vi "Entrenamiento Fuerza 4.vi"(8 "error in (no error)":errorcluster) -> (0 "error out":errorcluster, 3 "Message":string)   [LabVIEW 2014]
panel:
  in  "index":i32
  out "size(s)":i32
  out "Decorations[]":refnum<vi>[](array[refnum])
  out "Boolean":bool
  out "Impulso":string
  out "Tiempo Restante":string
  out "Time Target (s)":dbl=50.0
  out "Tiempo Transcurrido":string
  in  "Start":bool
  in  "Impulso":bool
  in  "Reset":bool
  in  "Back":bool
  in  "Help":bool
  in  "Slider":i32(slide) scale=0.0..100.0
  out "Horizontal Graduated Bar":i16(slide) scale=0.0..100.0
  in  "Remove Button":bool
  in  "Add Button":bool
  out "Opcional %":string="0%"
  in  "Opcional Bool":bool
  out "Biceps %":string="0%"
  in  "Biceps Bool":bool
  out "Pectorales %":string="0%"
  in  "Pectorales Bool":bool
  out "Trapecio %":string="0%"
  in  "Trapecio Bool":bool
  out "Dorsales %":string="0%"
  in  "Dorsales Bool":bool
  out "Lumbares %":string="0%"
  in  "Lumbares Bool":bool
  out "Abdomen %":string="0%"
  in  "Abdomen Bool":bool
  out "Gluteos %":string="0%"
  in  "Gluteos Bool":bool
  out "Isquiotibiales %":string="0%"
  in  "Isquiotibiales Bool":bool
  in  "Stop":bool
  out "Cuadríceps %":string="0%"
  in  "Cuadriceps Bool":bool
  out "date/time string":string="22/08/2015 01:25:29 a. m."
  # "Entrenamiento de Fuerza"
  # "Presentación"
  # "Seg"
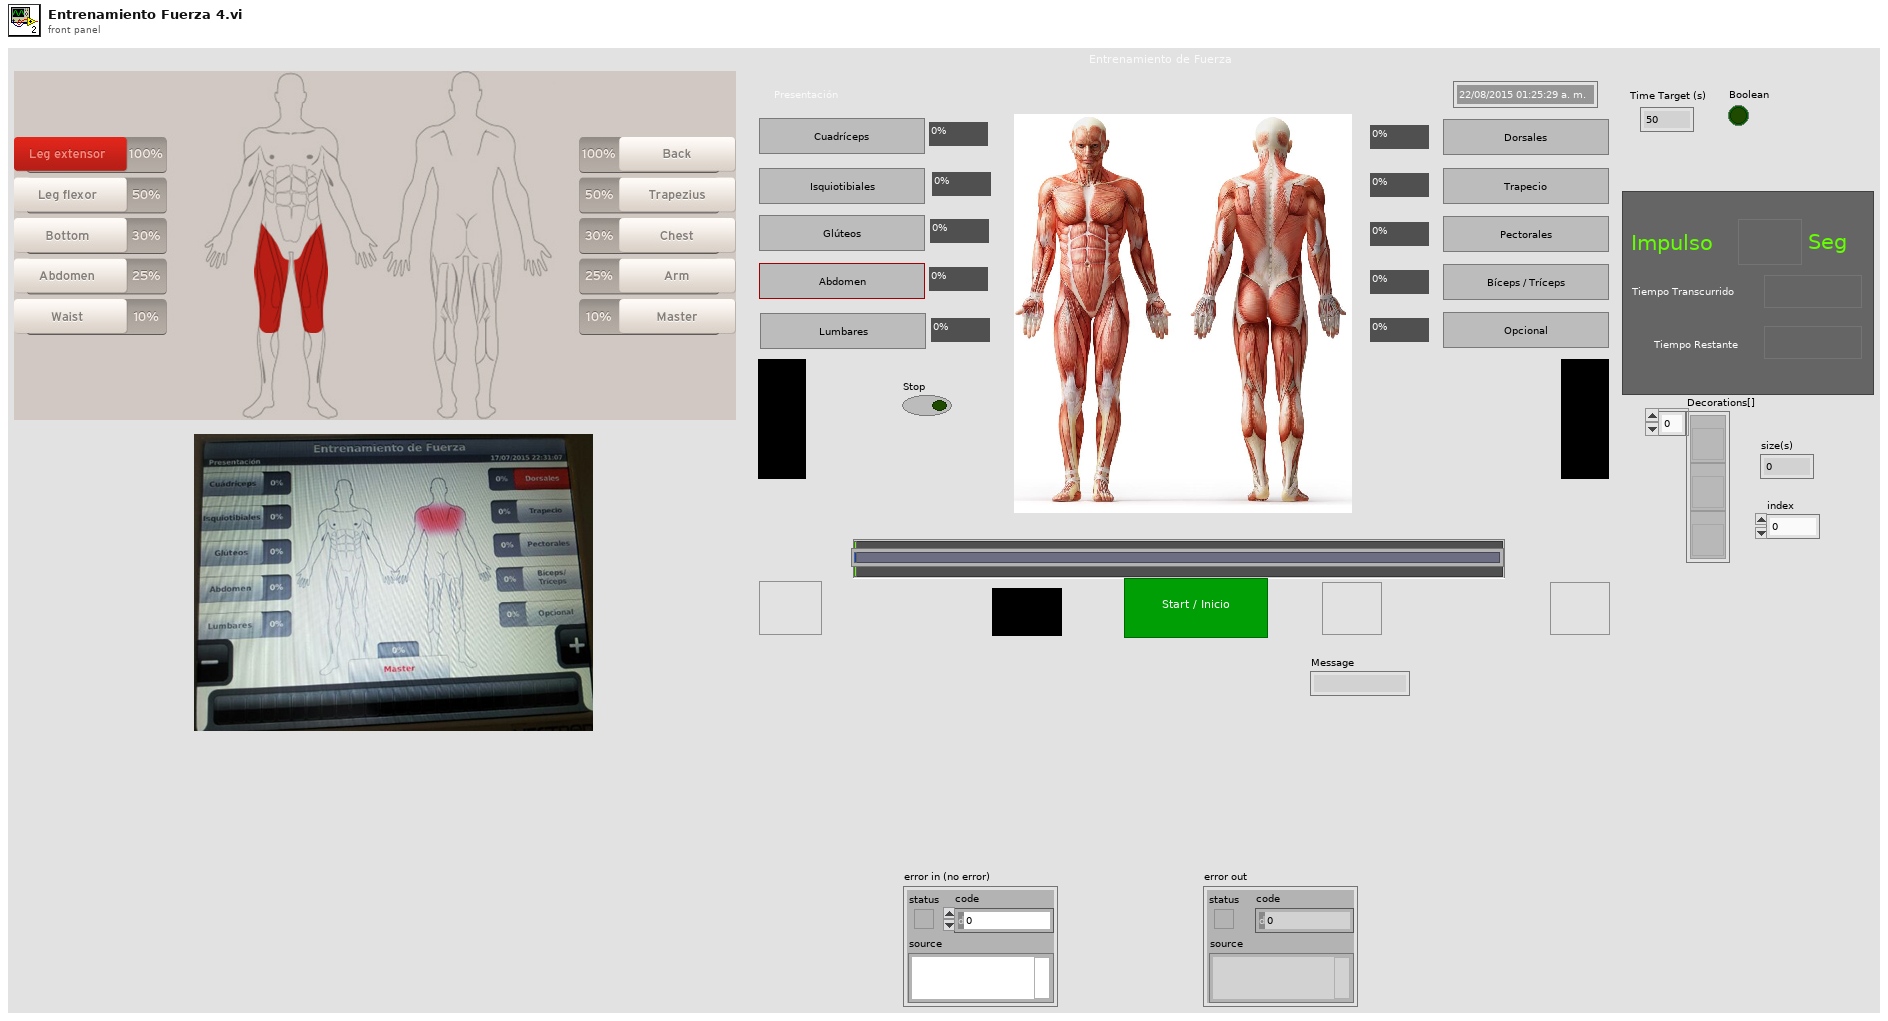
[diagram p1: front panel]
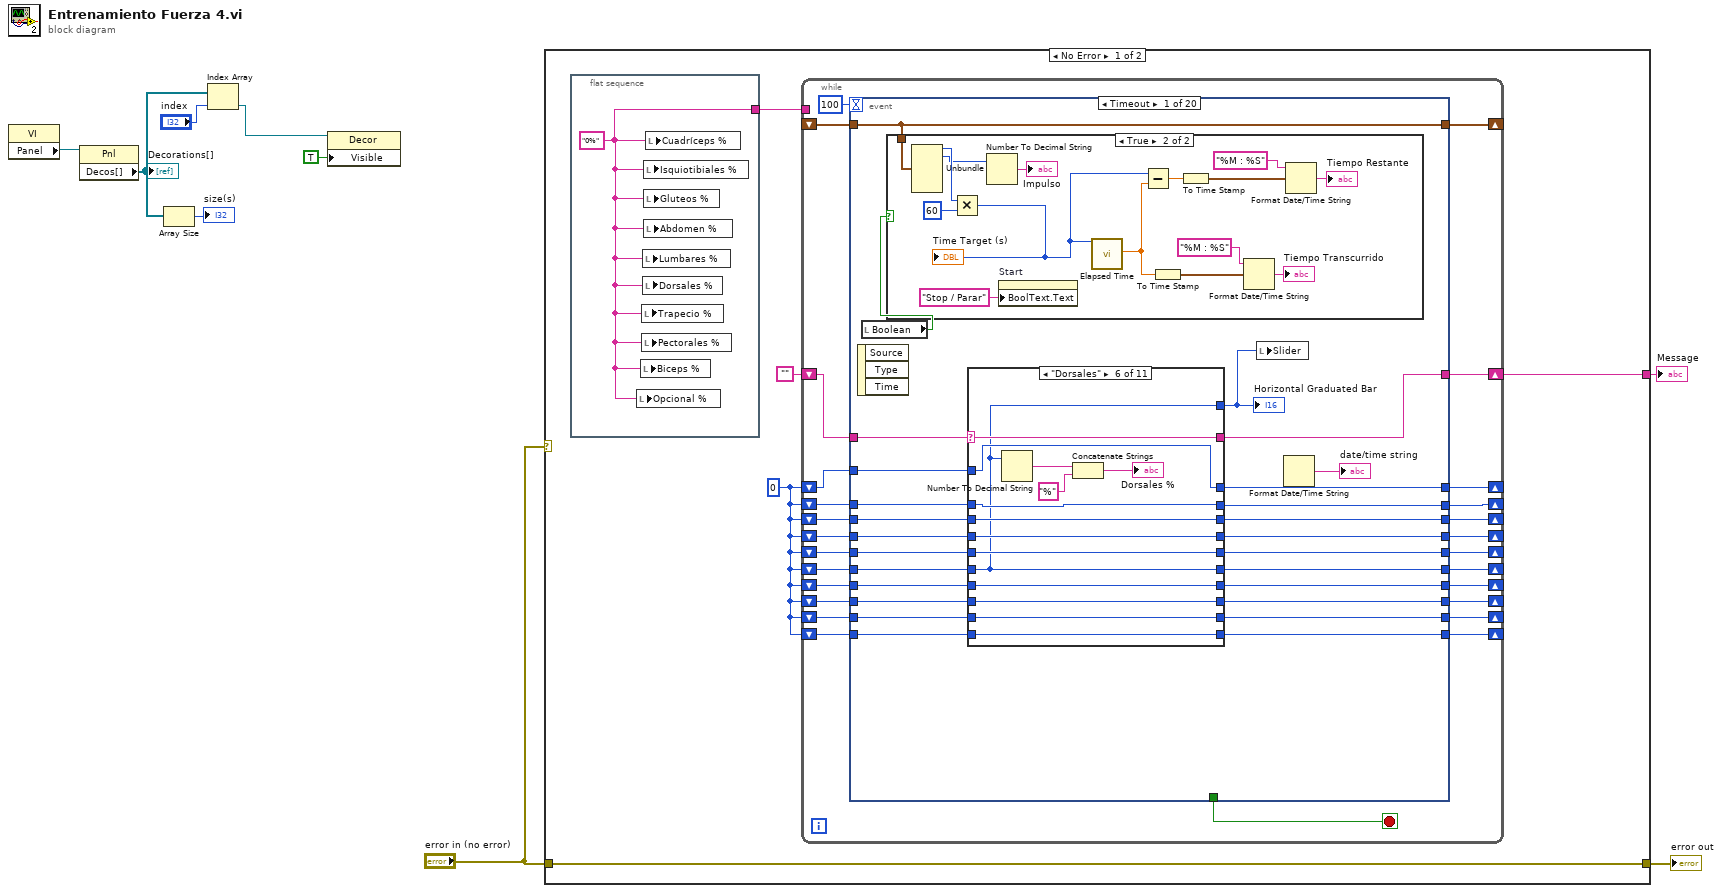
[diagram p0: block diagram]
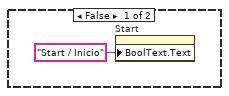
[diagram p2: hidden frame]
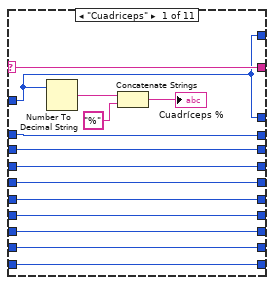
[diagram p3: hidden frame]
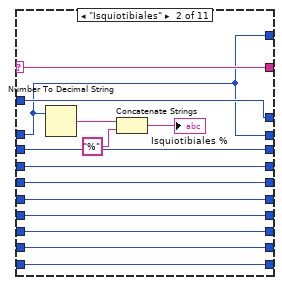
[diagram p4: hidden frame]
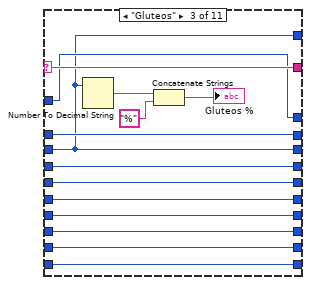
[diagram p5: hidden frame]
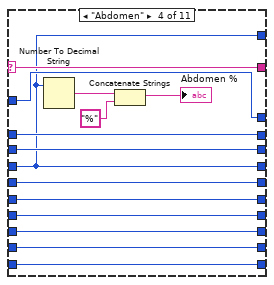
[diagram p6: hidden frame]
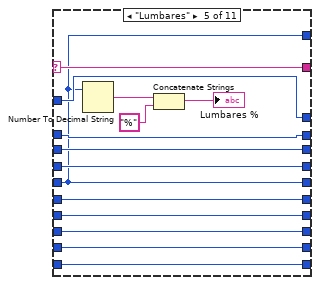
[diagram p7: hidden frame]
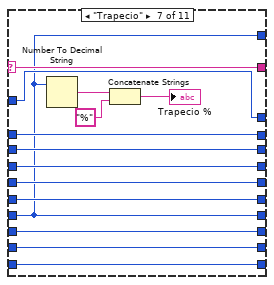
[diagram p8: hidden frame]
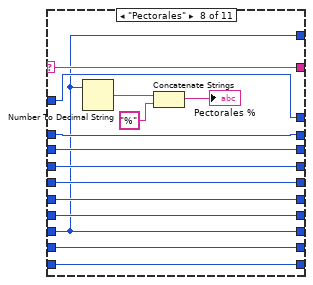
[diagram p9: hidden frame]
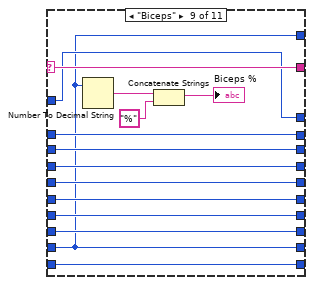
[diagram p10: hidden frame]
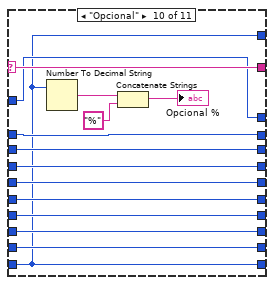
[diagram p11: hidden frame]
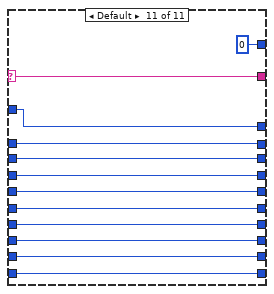
[diagram p12: hidden frame]
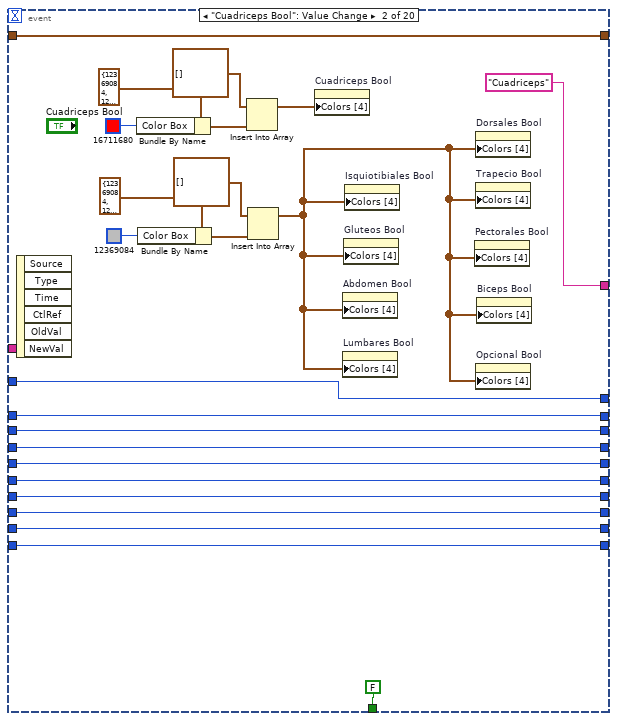
[diagram p13: hidden frame]
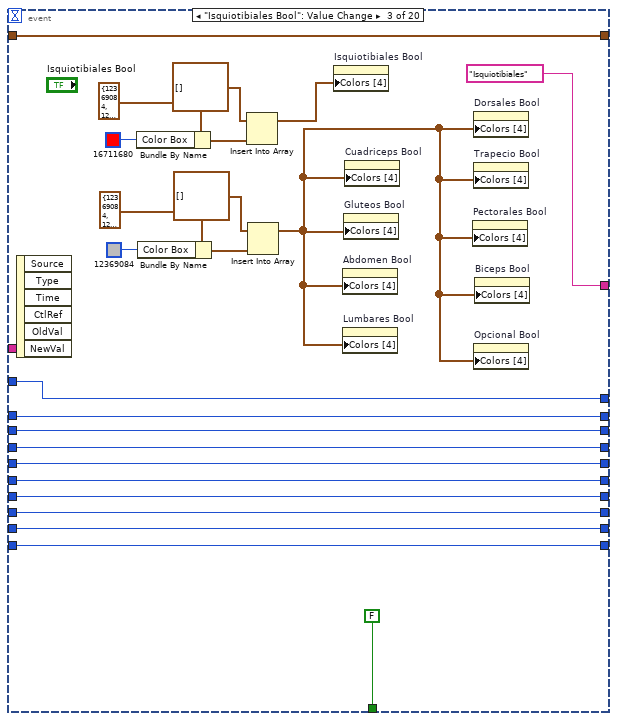
[diagram p14: hidden frame]
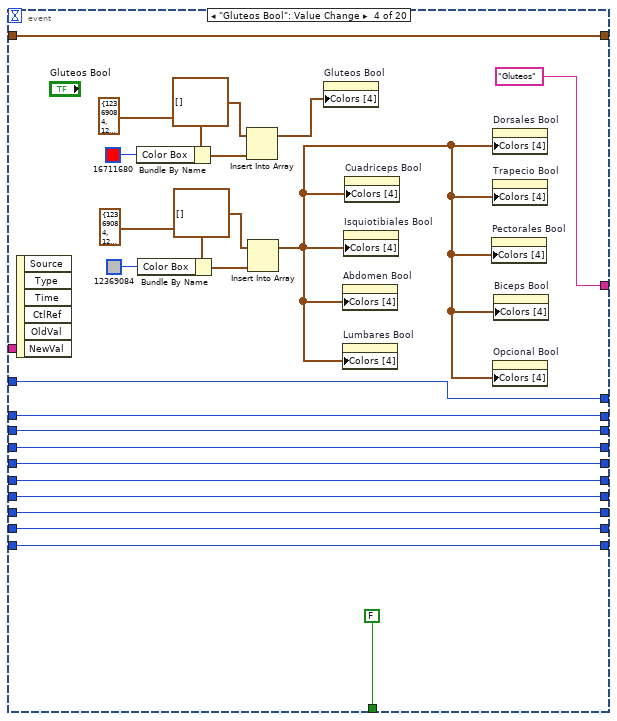
[diagram p15: hidden frame]
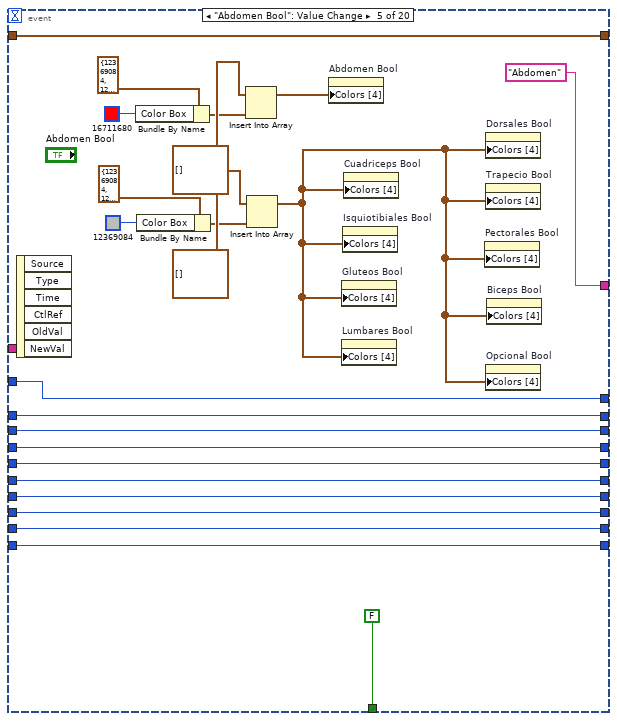
[diagram p16: hidden frame]
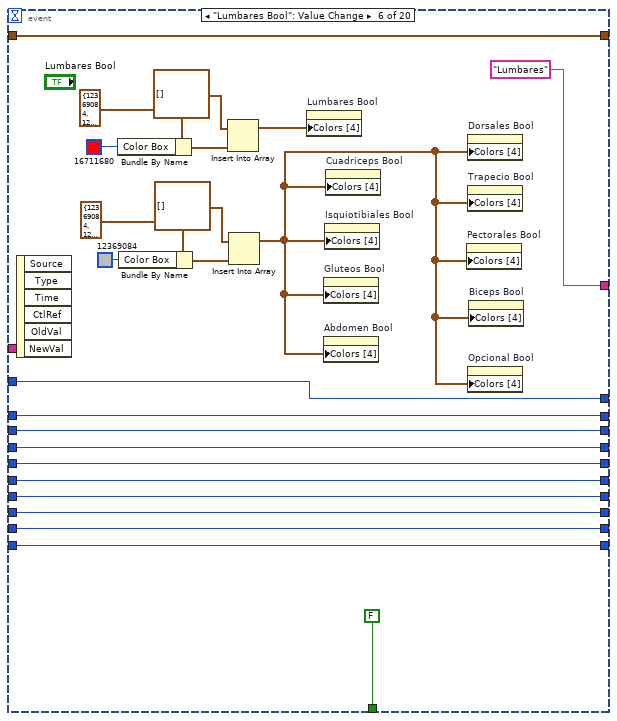
[diagram p17: hidden frame]
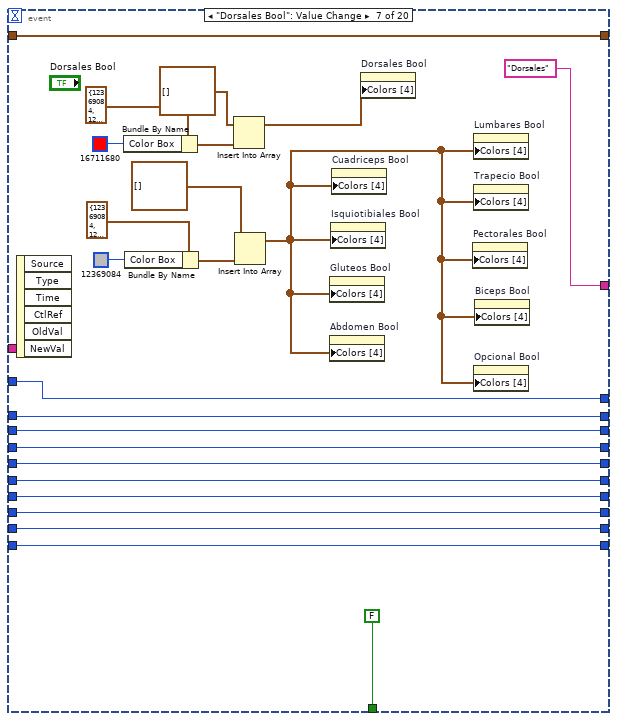
[diagram p18: hidden frame]
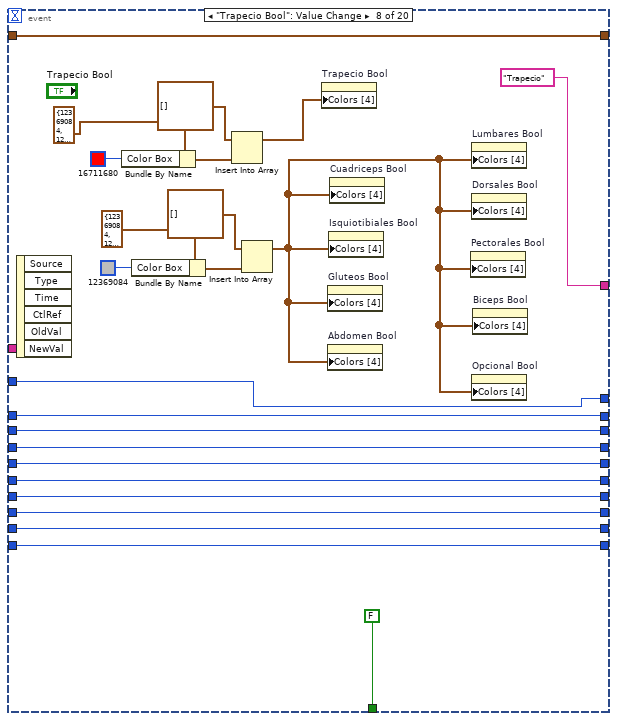
[diagram p19: hidden frame]
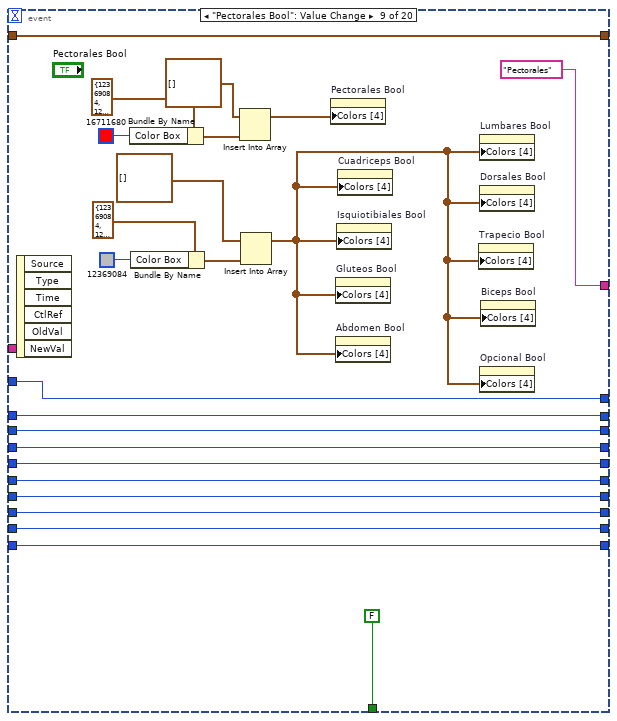
[diagram p20: hidden frame]
diagram:
  n1 = property class="VI"() -> ("Panel"=w6:refnum<vi>)  [unwired: 2 in, 2 out]
  n2 = property class="Pnl"(reference=w6) -> ("Decos[]"=w3:refnum<vi>[])  [unwired: 1 in, 2 out]
  "Decorations[]" <- w3
  n3 = Array Size(array=w3) -> (size(s)=→"size(s)":i32)
  n4 = Index Array(array=w3, index="index") -> (element=w2:refnum<vi>)
  n5 = property class="Decor"(reference=w2, "Visible"=TRUE) -> ()  [unwired: 1 in, 2 out]
  n6 = case shown="No Error" "error in (no error)" {
    tunnel: "error in (no error)" -> [w14 w1043]
    tunnel: [w14 w1043] -> w8
    tunnel: [w13 "Error" ("Message")] -> w7
    frame No Error {
      w11 = 0
      n7 = flat-sequence {
        tunnel: [w15] -> w10
        frame #0 {
          w15 = "0%" ("Cuadríceps %")
          n8 = local write "Opcional %"(w15) -> ()
          n9 = local write "Biceps %"(w15) -> ()
          n10 = local write "Trapecio %"(w15) -> ()
          n11 = local write "Pectorales %"(w15) -> ()
          n12 = local write "Lumbares %"(w15) -> ()
          n13 = local write "Dorsales %"(w15) -> ()
          n14 = local write "Isquiotibiales %"(w15) -> ()
          n15 = local write "Gluteos %"(w15) -> ()
          n16 = local write "Abdomen %"(w15) -> ()
          n17 = local write "Cuadríceps %"(w15) -> ()
        }
      }
      n18 = while {
        shift-right: [w39] -> w13
        shift-left: "" ("Message") -> [w38]
        shift-right: [w18] -> _
        shift-left: w11 -> [w37]
        shift-right: [w19] -> _
        shift-left: w11 -> [w36]
        shift-right: [w20] -> _
        shift-left: w11 -> [w35]
        shift-right: [w21] -> _
        shift-left: w11 -> [w34]
        shift-right: [w22] -> _
        shift-left: w11 -> [w33]
        shift-right: [w23] -> _
        shift-left: w11 -> [w32]
        shift-right: [w24] -> _
        shift-left: w11 -> [w31]
        shift-right: [w25] -> _
        shift-left: w11 -> [w30]
        shift-right: [w26] -> _
        shift-left: w11 -> [w29]
        shift-right: [w27] -> _
        shift-left: w11 -> [w28]
        tunnel: w10 -> [_]
        shift-right: [w16] -> _
        shift-left: _ -> [w17]
        stop <- w41 stop-if-true
        n19 = event shown="[0] Timeout" {
          selector: _ -> [_ _ _ _ _ _ _ _ _ _ _ _ _ _ _ _ _ _ _ _]
          dyn-events: _ -> [_ _ _ _ _ _ _ _ _ _ _ _ _ _ _ _ _ _ _ _]
          timeout: 100 -> [_ _ _ _ _ _ _ _ _ _ _ _ _ _ _ _ _ _ _ _]
          tunnel: [_ FALSE FALSE FALSE FALSE FALSE FALSE FALSE FALSE FALSE FALSE _ _ _ "Stop" TRUE ("Stop") FALSE ("Stop") TRUE ("Stop") FALSE ("Stop") _] -> w41
          tunnel: [w65 "Cuadriceps" ("Message") "Isquiotibiales" ("Message") "Gluteos" ("Message") "Abdomen" ("Message") "Lumbares" ("Message") "Dorsales" ("Message") "Trapecio" ("Message") "Pectorales" ("Message") "Biceps" ("Message") "Opcional" ("Message") w487 w689 w842 w984 "Back" ("Message") "Reset" ("Message") "Help" ("Message") "Impulso" ("Message") "Start" ("Message")] -> w39
          tunnel: w38 -> [w66 _ _ _ _ _ _ _ _ _ _ w487 w689 w842 w984 _ _ _ _ _]
          tunnel: w37 -> [w64 w237 w269 w283 w306 w329 w361 w384 w398 w430 w453 w486 w688 w843 w974 w989 _ w1006 w1019 w1032]
          tunnel: w36 -> [w63 w238 w268 w284 w307 w330 w360 w383 w407 w429 w452 w477 w679 w852 w975 w990 _ w1007 w1020 w1033]
          tunnel: w35 -> [w62 w239 w267 w285 w308 w331 w359 w382 w406 w428 w451 w478 w680 w851 w976 w991 _ w1008 w1021 w1034]
          tunnel: w34 -> [w61 w240 w266 w286 w309 w332 w358 w381 w405 w427 w450 w479 w681 w850 w977 w992 _ w1009 w1022 w1035]
          tunnel: w33 -> [w60 w241 w265 w287 w310 w333 w357 w380 w404 w426 w449 w480 w682 w849 w978 w993 _ w1010 w1023 w1036]
          tunnel: w32 -> [w59 w242 w264 w288 w311 w334 w356 w379 w403 w425 w448 w481 w683 w848 w979 w994 _ w1011 w1024 w1037]
          tunnel: w31 -> [w58 w243 w263 w289 w312 w335 w355 w378 w402 w424 w447 w482 w684 w847 w980 w995 _ w1012 w1025 w1038]
          tunnel: w30 -> [w45 w244 w262 w290 w313 w336 w354 w377 w401 w423 w446 w483 w685 w846 w981 w996 _ w1013 w1026 w1039]
          tunnel: w29 -> [w57 w245 w261 w291 w314 w337 w353 w376 w400 w422 w445 w484 w686 w845 w982 w997 _ w1014 w1027 w1040]
          tunnel: w28 -> [w56 w246 w260 w292 w315 w338 w352 w375 w399 w421 w444 w485 w687 w844 w983 w998 _ w1015 w1028 w1041]
          tunnel: [w55 w246 w260 w292 w315 w338 w352 w375 w399 w421 w444 w468 w670 w853 w983 w998 w1000 w1015 w1028 w1041] -> w27
          tunnel: [w54 w245 w261 w291 w314 w337 w353 w376 w400 w422 w445 w469 w671 w854 w982 w997 w1000 w1014 w1027 w1040] -> w26
          tunnel: [w53 w244 w262 w290 w313 w336 w354 w377 w401 w423 w446 w470 w672 w855 w981 w996 w1000 w1013 w1026 w1039] -> w25
          tunnel: [w52 w243 w263 w289 w312 w335 w355 w378 w402 w424 w447 w471 w673 w856 w980 w995 w1000 w1012 w1025 w1038] -> w24
          tunnel: [w51 w242 w264 w288 w311 w334 w356 w379 w403 w425 w448 w472 w674 w857 w979 w994 w1000 w1011 w1024 w1037] -> w23
          tunnel: [w50 w241 w265 w287 w310 w333 w357 w380 w404 w426 w449 w473 w675 w858 w978 w993 w1000 w1010 w1023 w1036] -> w22
          tunnel: [w49 w240 w266 w286 w309 w332 w358 w381 w405 w427 w450 w474 w676 w859 w977 w992 w1000 w1009 w1022 w1035] -> w21
          tunnel: [w48 w239 w267 w285 w308 w331 w359 w382 w406 w428 w451 w475 w677 w860 w976 w991 w1000 w1008 w1021 w1034] -> w20
          tunnel: [w47 w238 w268 w284 w307 w330 w360 w383 w407 w429 w452 w476 w678 w861 w975 w990 w1000 w1007 w1020 w1033] -> w19
          tunnel: [w46 w237 w269 w283 w306 w329 w361 w384 w398 w430 w453 w467 w669 w862 w974 w989 w1000 w1006 w1019 w1032] -> w18
          tunnel: w17 -> [w43 w236 w259 w282 w305 w328 w351 w374 w397 w420 w443 w466 w668 w840 w973 w986 w999 w1003 _ w1030]
          tunnel: [w43 w236 w259 w282 w305 w328 w351 w374 w397 w420 w443 w466 w668 w840 w973 w986 w999 w1003 w1016 w1030] -> w16
          event Timeout {
            n20 = event-data() -> ()  [unwired: 1 in, 3 out]
            n21 = local read "Boolean"() -> (w42:bool)
            n22 = case shown="True" w42 {
              tunnel: w43 -> [_ w73]
              frame False {
                n23 = property on="Start" class="Bool (strict)"("BoolText.Text"="Start / Inicio" ("Boolean Text.Text")) -> ()  [unwired: 2 in, 2 out]
              }
              frame True {
                n24 = Unbundle(w73) -> (w72:i32, w71:i32)  [unwired: 4 out]
                n25 = Multiply(x=w72, y=60) -> (x*y=w74:i32)
                "Time Target (s)" <- w74
                n26 = Number To Decimal String(number=w71) -> (decimal integer string=→"Impulso":string)  [unwired: 1 in]
                n27 = property on="Start" class="Bool (strict)"("BoolText.Text"="Stop / Parar" ("Boolean Text.Text")) -> ()  [unwired: 2 in, 2 out]
                n28 = call "Elapsed Time"("Time Target (s)"=w74) -> ("Elapsed Time (s)"=w80:dbl)  [unwired: 11 in, 7 out]
                n29 = Subtract(x=w74, y=w80) -> (x-y=w79:dbl)
                n30 = To Time Stamp(1:w80) -> (0:w81:timestamp)
                n31 = To Time Stamp(1:w79) -> (0:w76:timestamp)
                n32 = Format Date/Time String(time format string (%c)="%M : %S", seconds (now)=w81) -> (date/time string=→"Tiempo Transcurrido":string)  [unwired: 1 in]
                n33 = Format Date/Time String(time format string (%c)="%M : %S", seconds (now)=w76) -> (date/time string=→"Tiempo Restante":string)  [unwired: 1 in]
              }
            }
            n34 = case shown="\"Dorsales\"" w66 {
              selector: w66 -> [w97 w111 w125 w139 w153 w167 w181 w195 w209 w223 w235]
              tunnel: [w97 w111 w125 w139 w153 w167 w181 w195 w209 w223 w235] -> w65
              tunnel: w64 -> [w84 w99 w113 w127 w141 w155 w169 w183 w197 w212 w234]
              tunnel: w63 -> [w85 w98 w114 w128 w142 w156 w170 w184 w198 w211 w233]
              tunnel: w62 -> [w86 w100 w112 w129 w143 w161 w171 w185 w199 w213 w232]
              tunnel: w61 -> [w87 w101 w115 w126 w144 w162 w172 w191 w200 w214 w231]
              tunnel: w60 -> [w88 w102 w116 w130 w140 w163 w173 w190 w201 w215 w230]
              tunnel: w59 -> [w89 w103 w117 w131 w149 w154 w174 w189 w202 w216 w229]
              tunnel: w58 -> [w90 w104 w118 w132 w148 w160 w168 w188 w203 w217 w228]
              tunnel: w57 -> [w92 w106 w120 w134 w146 w158 w177 w187 w196 w219 w226]
              tunnel: w56 -> [w93 w107 w121 w135 w145 w157 w175 w186 w205 w210 w225]
              tunnel: [w93 w107 w121 w135 w145 w157 w175 w186 w205 w210 w225] -> w55
              tunnel: [w92 w106 w120 w134 w146 w158 w177 w187 w196 w219 w226] -> w54
              tunnel: [w91 w105 w119 w133 w147 w159 w176 w182 w204 w218 w227] -> w53
              tunnel: [w90 w104 w118 w132 w148 w160 w168 w188 w203 w217 w228] -> w52
              tunnel: [w89 w103 w117 w131 w149 w154 w174 w189 w202 w216 w229] -> w51
              tunnel: [w88 w102 w116 w130 w140 w163 w173 w190 w201 w215 w230] -> w50
              tunnel: [w87 w101 w115 w126 w144 w162 w172 w191 w200 w214 w231] -> w49
              tunnel: [w86 w100 w112 w129 w143 w161 w171 w185 w199 w213 w232] -> w48
              tunnel: [w85 w98 w114 w128 w142 w156 w170 w184 w198 w211 w233] -> w47
              tunnel: [w84 w99 w113 w127 w141 w155 w169 w183 w197 w212 w234] -> w46
              tunnel: w45 -> [w91 w105 w119 w133 w147 w159 w176 w182 w204 w218 w227]
              tunnel: [w84 w98 w112 w126 w140 w154 w168 w182 w196 w210 0] -> w44
              frame "Cuadriceps" {
                n35 = Number To Decimal String(number=w84) -> (decimal integer string=w96:string)  [unwired: 1 in]
                n36 = Concatenate Strings(w96, "%" ("string")) -> (→"Cuadríceps %":string)
              }
              frame "Isquiotibiales" {
                n37 = Number To Decimal String(number=w98) -> (decimal integer string=w110:string)  [unwired: 1 in]
                n38 = Concatenate Strings(w110, "%" ("string")) -> (→"Isquiotibiales %":string)
              }
              frame "Gluteos" {
                n39 = Number To Decimal String(number=w112) -> (decimal integer string=w124:string)  [unwired: 1 in]
                n40 = Concatenate Strings(w124, "%" ("string")) -> (→"Gluteos %":string)
              }
              frame "Abdomen" {
                n41 = Number To Decimal String(number=w126) -> (decimal integer string=w138:string)  [unwired: 1 in]
                n42 = Concatenate Strings(w138, "%" ("string")) -> (→"Abdomen %":string)
              }
              frame "Lumbares" {
                n43 = Number To Decimal String(number=w140) -> (decimal integer string=w152:string)  [unwired: 1 in]
                n44 = Concatenate Strings(w152, "%" ("string")) -> (→"Lumbares %":string)
              }
              frame "Dorsales" {
                n45 = Number To Decimal String(number=w154) -> (decimal integer string=w166:string)  [unwired: 1 in]
                n46 = Concatenate Strings(w166, "%" ("string")) -> (→"Dorsales %":string)
              }
              frame "Trapecio" {
                n47 = Number To Decimal String(number=w168) -> (decimal integer string=w180:string)  [unwired: 1 in]
                n48 = Concatenate Strings(w180, "%" ("string")) -> (→"Trapecio %":string)
              }
              frame "Pectorales" {
                n49 = Number To Decimal String(number=w182) -> (decimal integer string=w194:string)  [unwired: 1 in]
                n50 = Concatenate Strings(w194, "%" ("string")) -> (→"Pectorales %":string)
              }
              frame "Biceps" {
                n51 = Number To Decimal String(number=w196) -> (decimal integer string=w208:string)  [unwired: 1 in]
                n52 = Concatenate Strings(w208, "%" ("string")) -> (→"Biceps %":string)
              }
              frame "Opcional" {
                n53 = Number To Decimal String(number=w210) -> (decimal integer string=w222:string)  [unwired: 1 in]
                n54 = Concatenate Strings(w222, "%" ("string")) -> (→"Opcional %":string)
              }
              frame Default {
              }
            }
            "Horizontal Graduated Bar" <- w44
            n55 = local write "Slider"(w44) -> ()
            n56 = Format Date/Time String() -> (date/time string=→"date/time string":string)  [unwired: 3 in]
          }
          event "Cuadriceps Bool": Value Change {
            n57 = event-data() -> ()  [unwired: 1 in, 6 out]
            n58 = Bundle By Name(cluster=cluster{"Color Box":u32, "Color Box 2":u32} {"Color Box"=12369084, "Color Box 2"=12369084}, "Color Box"=u32 16711680 ("Color Box 2")) -> (w255:cluster{"Color Box":u32, "Color Box 2":u32})
            n59 = Bundle By Name(cluster=cluster{"Color Box":u32, "Color Box 2":u32} {"Color Box"=12369084, "Color Box 2"=12369084}, "Color Box"=u32 12369084 ("Color Box 2")) -> (w250:cluster{"Color Box":u32, "Color Box 2":u32})
            n60 = Insert Into Array(array=cluster{u32, u32}[] [] ("Colors [4]"), new element=w255) -> (w254:cluster{u32, u32}[])  [unwired: 1 in]
            n61 = Insert Into Array(array=cluster{u32, u32}[] [] ("Colors [4]"), new element=w250) -> (w248:cluster{u32, u32}[])  [unwired: 1 in]
            n62 = property on="Cuadriceps Bool" class="Bool"("Colors [4]"=w254) -> ()  [unwired: 2 in, 2 out]
            n63 = property on="Abdomen Bool" class="Bool"("Colors [4]"=w248) -> ()  [unwired: 2 in, 2 out]
            n64 = property on="Lumbares Bool" class="Bool"("Colors [4]"=w248) -> ()  [unwired: 2 in, 2 out]
            n65 = property on="Gluteos Bool" class="Bool"("Colors [4]"=w248) -> ()  [unwired: 2 in, 2 out]
            n66 = property on="Isquiotibiales Bool" class="Bool"("Colors [4]"=w248) -> ()  [unwired: 2 in, 2 out]
            n67 = property on="Pectorales Bool" class="Bool"("Colors [4]"=w248) -> ()  [unwired: 2 in, 2 out]
            n68 = property on="Dorsales Bool" class="Bool"("Colors [4]"=w248) -> ()  [unwired: 2 in, 2 out]
            n69 = property on="Trapecio Bool" class="Bool"("Colors [4]"=w248) -> ()  [unwired: 2 in, 2 out]
            n70 = property on="Opcional Bool" class="Bool"("Colors [4]"=w248) -> ()  [unwired: 2 in, 2 out]
            n71 = property on="Biceps Bool" class="Bool"("Colors [4]"=w248) -> ()  [unwired: 2 in, 2 out]
          }
          event "Isquiotibiales Bool": Value Change {
            n72 = event-data() -> ()  [unwired: 1 in, 6 out]
            n73 = Bundle By Name(cluster=cluster{"Color Box":u32, "Color Box 2":u32} {"Color Box"=12369084, "Color Box 2"=12369084}, "Color Box"=u32 16711680 ("Color Box 2")) -> (w277:cluster{"Color Box":u32, "Color Box 2":u32})
            n74 = Bundle By Name(cluster=cluster{"Color Box":u32, "Color Box 2":u32} {"Color Box"=12369084, "Color Box 2"=12369084}, "Color Box"=u32 12369084 ("Color Box 2")) -> (w273:cluster{"Color Box":u32, "Color Box 2":u32})
            n75 = Insert Into Array(array=cluster{u32, u32}[] [] ("Colors [4]"), new element=w277) -> (w271:cluster{u32, u32}[])  [unwired: 1 in]
            n76 = Insert Into Array(array=cluster{u32, u32}[] [] ("Colors [4]"), new element=w273) -> (w270:cluster{u32, u32}[])  [unwired: 1 in]
            n77 = property on="Isquiotibiales Bool" class="Bool"("Colors [4]"=w271) -> ()  [unwired: 2 in, 2 out]
            n78 = property on="Abdomen Bool" class="Bool"("Colors [4]"=w270) -> ()  [unwired: 2 in, 2 out]
            n79 = property on="Lumbares Bool" class="Bool"("Colors [4]"=w270) -> ()  [unwired: 2 in, 2 out]
            n80 = property on="Gluteos Bool" class="Bool"("Colors [4]"=w270) -> ()  [unwired: 2 in, 2 out]
            n81 = property on="Cuadriceps Bool" class="Bool"("Colors [4]"=w270) -> ()  [unwired: 2 in, 2 out]
            n82 = property on="Pectorales Bool" class="Bool"("Colors [4]"=w270) -> ()  [unwired: 2 in, 2 out]
            n83 = property on="Dorsales Bool" class="Bool"("Colors [4]"=w270) -> ()  [unwired: 2 in, 2 out]
            n84 = property on="Trapecio Bool" class="Bool"("Colors [4]"=w270) -> ()  [unwired: 2 in, 2 out]
            n85 = property on="Opcional Bool" class="Bool"("Colors [4]"=w270) -> ()  [unwired: 2 in, 2 out]
            n86 = property on="Biceps Bool" class="Bool"("Colors [4]"=w270) -> ()  [unwired: 2 in, 2 out]
          }
          event "Gluteos Bool": Value Change {
            n87 = event-data() -> ()  [unwired: 1 in, 6 out]
            n88 = Bundle By Name(cluster=cluster{"Color Box":u32, "Color Box 2":u32} {"Color Box"=12369084, "Color Box 2"=12369084}, "Color Box"=u32 16711680 ("Color Box 2")) -> (w300:cluster{"Color Box":u32, "Color Box 2":u32})
            n89 = Bundle By Name(cluster=cluster{"Color Box":u32, "Color Box 2":u32} {"Color Box"=12369084, "Color Box 2"=12369084}, "Color Box"=u32 12369084 ("Color Box 2")) -> (w296:cluster{"Color Box":u32, "Color Box 2":u32})
            n90 = Insert Into Array(array=cluster{u32, u32}[] [] ("Colors [4]"), new element=w300) -> (w294:cluster{u32, u32}[])  [unwired: 1 in]
            n91 = Insert Into Array(array=cluster{u32, u32}[] [] ("Colors [4]"), new element=w296) -> (w293:cluster{u32, u32}[])  [unwired: 1 in]
            n92 = property on="Gluteos Bool" class="Bool"("Colors [4]"=w294) -> ()  [unwired: 2 in, 2 out]
            n93 = property on="Abdomen Bool" class="Bool"("Colors [4]"=w293) -> ()  [unwired: 2 in, 2 out]
            n94 = property on="Lumbares Bool" class="Bool"("Colors [4]"=w293) -> ()  [unwired: 2 in, 2 out]
            n95 = property on="Isquiotibiales Bool" class="Bool"("Colors [4]"=w293) -> ()  [unwired: 2 in, 2 out]
            n96 = property on="Cuadriceps Bool" class="Bool"("Colors [4]"=w293) -> ()  [unwired: 2 in, 2 out]
            n97 = property on="Pectorales Bool" class="Bool"("Colors [4]"=w293) -> ()  [unwired: 2 in, 2 out]
            n98 = property on="Dorsales Bool" class="Bool"("Colors [4]"=w293) -> ()  [unwired: 2 in, 2 out]
            n99 = property on="Trapecio Bool" class="Bool"("Colors [4]"=w293) -> ()  [unwired: 2 in, 2 out]
            n100 = property on="Opcional Bool" class="Bool"("Colors [4]"=w293) -> ()  [unwired: 2 in, 2 out]
            n101 = property on="Biceps Bool" class="Bool"("Colors [4]"=w293) -> ()  [unwired: 2 in, 2 out]
          }
          event "Abdomen Bool": Value Change {
            n102 = event-data() -> ()  [unwired: 1 in, 6 out]
            n103 = Bundle By Name(cluster=cluster{"Color Box":u32, "Color Box 2":u32} {"Color Box"=12369084, "Color Box 2"=12369084}, "Color Box"=u32 16711680 ("Color Box 2")) -> (w323:cluster{"Color Box":u32, "Color Box 2":u32})
            n104 = Bundle By Name(cluster=cluster{"Color Box":u32, "Color Box 2":u32} {"Color Box"=12369084, "Color Box 2"=12369084}, "Color Box"=u32 12369084 ("Color Box 2")) -> (w319:cluster{"Color Box":u32, "Color Box 2":u32})
            n105 = Insert Into Array(array=cluster{u32, u32}[] [] ("Colors [4]"), new element=w323) -> (w317:cluster{u32, u32}[])  [unwired: 1 in]
            n106 = Insert Into Array(array=cluster{u32, u32}[] [] ("Colors [4]"), new element=w319) -> (w316:cluster{u32, u32}[])  [unwired: 1 in]
            n107 = property on="Abdomen Bool" class="Bool"("Colors [4]"=w317) -> ()  [unwired: 2 in, 2 out]
            n108 = property on="Gluteos Bool" class="Bool"("Colors [4]"=w316) -> ()  [unwired: 2 in, 2 out]
            n109 = property on="Lumbares Bool" class="Bool"("Colors [4]"=w316) -> ()  [unwired: 2 in, 2 out]
            n110 = property on="Isquiotibiales Bool" class="Bool"("Colors [4]"=w316) -> ()  [unwired: 2 in, 2 out]
            n111 = property on="Cuadriceps Bool" class="Bool"("Colors [4]"=w316) -> ()  [unwired: 2 in, 2 out]
            n112 = property on="Pectorales Bool" class="Bool"("Colors [4]"=w316) -> ()  [unwired: 2 in, 2 out]
            n113 = property on="Dorsales Bool" class="Bool"("Colors [4]"=w316) -> ()  [unwired: 2 in, 2 out]
            n114 = property on="Trapecio Bool" class="Bool"("Colors [4]"=w316) -> ()  [unwired: 2 in, 2 out]
            n115 = property on="Opcional Bool" class="Bool"("Colors [4]"=w316) -> ()  [unwired: 2 in, 2 out]
            n116 = property on="Biceps Bool" class="Bool"("Colors [4]"=w316) -> ()  [unwired: 2 in, 2 out]
          }
          event "Lumbares Bool": Value Change {
            n117 = event-data() -> ()  [unwired: 1 in, 6 out]
            n118 = Bundle By Name(cluster=cluster{"Color Box":u32, "Color Box 2":u32} {"Color Box"=12369084, "Color Box 2"=12369084}, "Color Box"=u32 16711680 ("Color Box 2")) -> (w346:cluster{"Color Box":u32, "Color Box 2":u32})
            n119 = Bundle By Name(cluster=cluster{"Color Box":u32, "Color Box 2":u32} {"Color Box"=12369084, "Color Box 2"=12369084}, "Color Box"=u32 12369084 ("Color Box 2")) -> (w342:cluster{"Color Box":u32, "Color Box 2":u32})
            n120 = Insert Into Array(array=cluster{u32, u32}[] [] ("Colors [4]"), new element=w346) -> (w340:cluster{u32, u32}[])  [unwired: 1 in]
            n121 = Insert Into Array(array=cluster{u32, u32}[] [] ("Colors [4]"), new element=w342) -> (w339:cluster{u32, u32}[])  [unwired: 1 in]
            n122 = property on="Lumbares Bool" class="Bool"("Colors [4]"=w340) -> ()  [unwired: 2 in, 2 out]
            n123 = property on="Gluteos Bool" class="Bool"("Colors [4]"=w339) -> ()  [unwired: 2 in, 2 out]
            n124 = property on="Abdomen Bool" class="Bool"("Colors [4]"=w339) -> ()  [unwired: 2 in, 2 out]
            n125 = property on="Isquiotibiales Bool" class="Bool"("Colors [4]"=w339) -> ()  [unwired: 2 in, 2 out]
            n126 = property on="Cuadriceps Bool" class="Bool"("Colors [4]"=w339) -> ()  [unwired: 2 in, 2 out]
            n127 = property on="Pectorales Bool" class="Bool"("Colors [4]"=w339) -> ()  [unwired: 2 in, 2 out]
            n128 = property on="Dorsales Bool" class="Bool"("Colors [4]"=w339) -> ()  [unwired: 2 in, 2 out]
            n129 = property on="Trapecio Bool" class="Bool"("Colors [4]"=w339) -> ()  [unwired: 2 in, 2 out]
            n130 = property on="Opcional Bool" class="Bool"("Colors [4]"=w339) -> ()  [unwired: 2 in, 2 out]
            n131 = property on="Biceps Bool" class="Bool"("Colors [4]"=w339) -> ()  [unwired: 2 in, 2 out]
          }
          event "Dorsales Bool": Value Change {
            n132 = event-data() -> ()  [unwired: 1 in, 6 out]
            n133 = Bundle By Name(cluster=cluster{"Color Box":u32, "Color Box 2":u32} {"Color Box"=12369084, "Color Box 2"=12369084}, "Color Box"=u32 16711680 ("Color Box 2")) -> (w369:cluster{"Color Box":u32, "Color Box 2":u32})
            n134 = Bundle By Name(cluster=cluster{"Color Box":u32, "Color Box 2":u32} {"Color Box"=12369084, "Color Box 2"=12369084}, "Color Box"=u32 12369084 ("Color Box 2")) -> (w365:cluster{"Color Box":u32, "Color Box 2":u32})
            n135 = Insert Into Array(array=cluster{u32, u32}[] [] ("Colors [4]"), new element=w369) -> (w362:cluster{u32, u32}[])  [unwired: 1 in]
            n136 = Insert Into Array(array=cluster{u32, u32}[] [] ("Colors [4]"), new element=w365) -> (w363:cluster{u32, u32}[])  [unwired: 1 in]
            n137 = property on="Gluteos Bool" class="Bool"("Colors [4]"=w363) -> ()  [unwired: 2 in, 2 out]
            n138 = property on="Abdomen Bool" class="Bool"("Colors [4]"=w363) -> ()  [unwired: 2 in, 2 out]
            n139 = property on="Isquiotibiales Bool" class="Bool"("Colors [4]"=w363) -> ()  [unwired: 2 in, 2 out]
            n140 = property on="Cuadriceps Bool" class="Bool"("Colors [4]"=w363) -> ()  [unwired: 2 in, 2 out]
            n141 = property on="Dorsales Bool" class="Bool"("Colors [4]"=w362) -> ()  [unwired: 2 in, 2 out]
            n142 = property on="Pectorales Bool" class="Bool"("Colors [4]"=w363) -> ()  [unwired: 2 in, 2 out]
            n143 = property on="Lumbares Bool" class="Bool"("Colors [4]"=w363) -> ()  [unwired: 2 in, 2 out]
            n144 = property on="Trapecio Bool" class="Bool"("Colors [4]"=w363) -> ()  [unwired: 2 in, 2 out]
            n145 = property on="Opcional Bool" class="Bool"("Colors [4]"=w363) -> ()  [unwired: 2 in, 2 out]
            n146 = property on="Biceps Bool" class="Bool"("Colors [4]"=w363) -> ()  [unwired: 2 in, 2 out]
          }
          event "Trapecio Bool": Value Change {
            n147 = event-data() -> ()  [unwired: 1 in, 6 out]
            n148 = Bundle By Name(cluster=cluster{"Color Box":u32, "Color Box 2":u32} {"Color Box"=12369084, "Color Box 2"=12369084}, "Color Box"=u32 16711680 ("Color Box 2")) -> (w392:cluster{"Color Box":u32, "Color Box 2":u32})
            n149 = Bundle By Name(cluster=cluster{"Color Box":u32, "Color Box 2":u32} {"Color Box"=12369084, "Color Box 2"=12369084}, "Color Box"=u32 12369084 ("Color Box 2")) -> (w388:cluster{"Color Box":u32, "Color Box 2":u32})
            n150 = Insert Into Array(array=cluster{u32, u32}[] [] ("Colors [4]"), new element=w392) -> (w385:cluster{u32, u32}[])  [unwired: 1 in]
            n151 = Insert Into Array(array=cluster{u32, u32}[] [] ("Colors [4]"), new element=w388) -> (w386:cluster{u32, u32}[])  [unwired: 1 in]
            n152 = property on="Trapecio Bool" class="Bool"("Colors [4]"=w385) -> ()  [unwired: 2 in, 2 out]
            n153 = property on="Gluteos Bool" class="Bool"("Colors [4]"=w386) -> ()  [unwired: 2 in, 2 out]
            n154 = property on="Abdomen Bool" class="Bool"("Colors [4]"=w386) -> ()  [unwired: 2 in, 2 out]
            n155 = property on="Isquiotibiales Bool" class="Bool"("Colors [4]"=w386) -> ()  [unwired: 2 in, 2 out]
            n156 = property on="Cuadriceps Bool" class="Bool"("Colors [4]"=w386) -> ()  [unwired: 2 in, 2 out]
            n157 = property on="Pectorales Bool" class="Bool"("Colors [4]"=w386) -> ()  [unwired: 2 in, 2 out]
            n158 = property on="Lumbares Bool" class="Bool"("Colors [4]"=w386) -> ()  [unwired: 2 in, 2 out]
            n159 = property on="Dorsales Bool" class="Bool"("Colors [4]"=w386) -> ()  [unwired: 2 in, 2 out]
            n160 = property on="Opcional Bool" class="Bool"("Colors [4]"=w386) -> ()  [unwired: 2 in, 2 out]
            n161 = property on="Biceps Bool" class="Bool"("Colors [4]"=w386) -> ()  [unwired: 2 in, 2 out]
          }
          event "Pectorales Bool": Value Change {
            n162 = event-data() -> ()  [unwired: 1 in, 6 out]
            n163 = Bundle By Name(cluster=cluster{"Color Box":u32, "Color Box 2":u32} {"Color Box"=12369084, "Color Box 2"=12369084}, "Color Box"=u32 16711680 ("Color Box 2")) -> (w415:cluster{"Color Box":u32, "Color Box 2":u32})
            n164 = Bundle By Name(cluster=cluster{"Color Box":u32, "Color Box 2":u32} {"Color Box"=12369084, "Color Box 2"=12369084}, "Color Box"=u32 12369084 ("Color Box 2")) -> (w411:cluster{"Color Box":u32, "Color Box 2":u32})
            n165 = Insert Into Array(array=cluster{u32, u32}[] [] ("Colors [4]"), new element=w415) -> (w408:cluster{u32, u32}[])  [unwired: 1 in]
            n166 = Insert Into Array(array=cluster{u32, u32}[] [] ("Colors [4]"), new element=w411) -> (w409:cluster{u32, u32}[])  [unwired: 1 in]
            n167 = property on="Pectorales Bool" class="Bool"("Colors [4]"=w408) -> ()  [unwired: 2 in, 2 out]
            n168 = property on="Gluteos Bool" class="Bool"("Colors [4]"=w409) -> ()  [unwired: 2 in, 2 out]
            n169 = property on="Abdomen Bool" class="Bool"("Colors [4]"=w409) -> ()  [unwired: 2 in, 2 out]
            n170 = property on="Isquiotibiales Bool" class="Bool"("Colors [4]"=w409) -> ()  [unwired: 2 in, 2 out]
            n171 = property on="Cuadriceps Bool" class="Bool"("Colors [4]"=w409) -> ()  [unwired: 2 in, 2 out]
            n172 = property on="Trapecio Bool" class="Bool"("Colors [4]"=w409) -> ()  [unwired: 2 in, 2 out]
            n173 = property on="Lumbares Bool" class="Bool"("Colors [4]"=w409) -> ()  [unwired: 2 in, 2 out]
            n174 = property on="Dorsales Bool" class="Bool"("Colors [4]"=w409) -> ()  [unwired: 2 in, 2 out]
            n175 = property on="Opcional Bool" class="Bool"("Colors [4]"=w409) -> ()  [unwired: 2 in, 2 out]
            n176 = property on="Biceps Bool" class="Bool"("Colors [4]"=w409) -> ()  [unwired: 2 in, 2 out]
          }
          event "Biceps Bool": Value Change {
            n177 = event-data() -> ()  [unwired: 1 in, 6 out]
            n178 = Bundle By Name(cluster=cluster{"Color Box":u32, "Color Box 2":u32} {"Color Box"=12369084, "Color Box 2"=12369084}, "Color Box"=u32 16711680 ("Color Box 2")) -> (w439:cluster{"Color Box":u32, "Color Box 2":u32})
            n179 = Bundle By Name(cluster=cluster{"Color Box":u32, "Color Box 2":u32} {"Color Box"=12369084, "Color Box 2"=12369084}, "Color Box"=u32 12369084 ("Color Box 2")) -> (w435:cluster{"Color Box":u32, "Color Box 2":u32})
            n180 = Insert Into Array(array=cluster{u32, u32}[] [] ("Colors [4]"), new element=w439) -> (w432:cluster{u32, u32}[])  [unwired: 1 in]
            n181 = Insert Into Array(array=cluster{u32, u32}[] [] ("Colors [4]"), new element=w435) -> (w433:cluster{u32, u32}[])  [unwired: 1 in]
            n182 = property on="Biceps Bool" class="Bool"("Colors [4]"=w432) -> ()  [unwired: 2 in, 2 out]
            n183 = property on="Gluteos Bool" class="Bool"("Colors [4]"=w433) -> ()  [unwired: 2 in, 2 out]
            n184 = property on="Abdomen Bool" class="Bool"("Colors [4]"=w433) -> ()  [unwired: 2 in, 2 out]
            n185 = property on="Isquiotibiales Bool" class="Bool"("Colors [4]"=w433) -> ()  [unwired: 2 in, 2 out]
            n186 = property on="Cuadriceps Bool" class="Bool"("Colors [4]"=w433) -> ()  [unwired: 2 in, 2 out]
            n187 = property on="Trapecio Bool" class="Bool"("Colors [4]"=w433) -> ()  [unwired: 2 in, 2 out]
            n188 = property on="Lumbares Bool" class="Bool"("Colors [4]"=w433) -> ()  [unwired: 2 in, 2 out]
            n189 = property on="Dorsales Bool" class="Bool"("Colors [4]"=w433) -> ()  [unwired: 2 in, 2 out]
            n190 = property on="Opcional Bool" class="Bool"("Colors [4]"=w433) -> ()  [unwired: 2 in, 2 out]
            n191 = property on="Pectorales Bool" class="Bool"("Colors [4]"=w433) -> ()  [unwired: 2 in, 2 out]
          }
          event "Opcional Bool": Value Change {
            n192 = event-data() -> ()  [unwired: 1 in, 6 out]
            n193 = Bundle By Name(cluster=cluster{"Color Box":u32, "Color Box 2":u32} {"Color Box"=12369084, "Color Box 2"=12369084}, "Color Box"=u32 16711680 ("Color Box 2")) -> (w461:cluster{"Color Box":u32, "Color Box 2":u32})
            n194 = Bundle By Name(cluster=cluster{"Color Box":u32, "Color Box 2":u32} {"Color Box"=12369084, "Color Box 2"=12369084}, "Color Box"=u32 12369084 ("Color Box 2")) -> (w457:cluster{"Color Box":u32, "Color Box 2":u32})
            n195 = Insert Into Array(array=cluster{u32, u32}[] [] ("Colors [4]"), new element=w461) -> (w454:cluster{u32, u32}[])  [unwired: 1 in]
            n196 = Insert Into Array(array=cluster{u32, u32}[] [] ("Colors [4]"), new element=w457) -> (w455:cluster{u32, u32}[])  [unwired: 1 in]
            n197 = property on="Opcional Bool" class="Bool"("Colors [4]"=w454) -> ()  [unwired: 2 in, 2 out]
            n198 = property on="Gluteos Bool" class="Bool"("Colors [4]"=w455) -> ()  [unwired: 2 in, 2 out]
            n199 = property on="Abdomen Bool" class="Bool"("Colors [4]"=w455) -> ()  [unwired: 2 in, 2 out]
            n200 = property on="Isquiotibiales Bool" class="Bool"("Colors [4]"=w455) -> ()  [unwired: 2 in, 2 out]
            n201 = property on="Cuadriceps Bool" class="Bool"("Colors [4]"=w455) -> ()  [unwired: 2 in, 2 out]
            n202 = property on="Trapecio Bool" class="Bool"("Colors [4]"=w455) -> ()  [unwired: 2 in, 2 out]
            n203 = property on="Lumbares Bool" class="Bool"("Colors [4]"=w455) -> ()  [unwired: 2 in, 2 out]
            n204 = property on="Dorsales Bool" class="Bool"("Colors [4]"=w455) -> ()  [unwired: 2 in, 2 out]
            n205 = property on="Biceps Bool" class="Bool"("Colors [4]"=w455) -> ()  [unwired: 2 in, 2 out]
            n206 = property on="Pectorales Bool" class="Bool"("Colors [4]"=w455) -> ()  [unwired: 2 in, 2 out]
          }
          event "Add Button": Value Change {
            n207 = event-data() -> ()  [unwired: 1 in, 6 out]
            n208 = case shown="\"Pectorales\"" w487 {
              tunnel: w486 -> [w498 w507 w525 w543 w561 w579 w597 w615 w633 w651 w667]
              tunnel: w485 -> [w497 w515 w532 w549 w566 w583 w600 w617 w634 w642 w658]
              tunnel: w484 -> [w496 w514 w531 w548 w565 w582 w599 w616 w624 w643 w659]
              tunnel: w483 -> [w495 w513 w530 w547 w564 w581 w598 w609 w626 w644 w660]
              tunnel: w482 -> [w494 w512 w529 w546 w563 w580 w591 w608 w627 w645 w661]
              tunnel: w481 -> [w493 w511 w528 w545 w562 w573 w592 w610 w628 w646 w662]
              tunnel: w480 -> [w492 w510 w527 w544 w557 w575 w593 w611 w629 w647 w663]
              tunnel: w479 -> [w491 w509 w526 w540 w558 w576 w594 w612 w630 w648 w664]
              tunnel: w478 -> [w490 w508 w523 w541 w559 w577 w595 w613 w631 w649 w665]
              tunnel: w477 -> [w489 w506 w524 w542 w560 w578 w596 w614 w632 w650 w666]
              tunnel: [w497 w515 w532 w549 w566 w583 w600 w617 w634 w641 w658] -> w468
              tunnel: [w496 w514 w531 w548 w565 w582 w599 w616 w625 w643 w659] -> w469
              tunnel: [w495 w513 w530 w547 w564 w581 w598 w607 w626 w644 w660] -> w470
              tunnel: [w494 w512 w529 w546 w563 w580 w590 w608 w627 w645 w661] -> w471
              tunnel: [w493 w511 w528 w545 w562 w574 w592 w610 w628 w646 w662] -> w472
              tunnel: [w492 w510 w527 w544 w556 w575 w593 w611 w629 w647 w663] -> w473
              tunnel: [w491 w509 w526 w539 w558 w576 w594 w612 w630 w648 w664] -> w474
              tunnel: [w490 w508 w522 w541 w559 w577 w595 w613 w631 w649 w665] -> w475
              tunnel: [w489 w505 w524 w542 w560 w578 w596 w614 w632 w650 w666] -> w476
              tunnel: [w488 w507 w525 w543 w561 w579 w597 w615 w633 w651 w667] -> w467
              frame "Cuadriceps" {
                n209 = Greater Or Equal To 0?(x=w498) -> (x >= 0?=w502:bool)
                n210 = Less Or Equal?(x=w498, y=100) -> (x <= y?=w500:bool)
                n211 = Add(x=w498, y=5) -> (x+y=w504:i32)
                n212 = And(x=w502, y=w500) -> (x .and. y?=w501:bool)
                n213 = Select(t=w504, s=w501, f=w498) -> (s? t:f=w488:i32)
              }
              frame "Isquiotibiales" {
                n214 = Greater Or Equal To 0?(x=w506) -> (x >= 0?=w519:bool)
                n215 = Less Or Equal?(x=w506, y=100) -> (x <= y?=w517:bool)
                n216 = Add(x=w506, y=5) -> (x+y=w521:i32)
                n217 = And(x=w519, y=w517) -> (x .and. y?=w518:bool)
                n218 = Select(t=w521, s=w518, f=w506) -> (s? t:f=w505:i32)
              }
              frame "Gluteos" {
                n219 = Greater Or Equal To 0?(x=w523) -> (x >= 0?=w536:bool)
                n220 = Less Or Equal?(x=w523, y=100) -> (x <= y?=w534:bool)
                n221 = Add(x=w523, y=5) -> (x+y=w538:i32)
                n222 = And(x=w536, y=w534) -> (x .and. y?=w535:bool)
                n223 = Select(t=w538, s=w535, f=w523) -> (s? t:f=w522:i32)
              }
              frame "Abdomen" {
                n224 = Greater Or Equal To 0?(x=w540) -> (x >= 0?=w553:bool)
                n225 = Less Or Equal?(x=w540, y=100) -> (x <= y?=w551:bool)
                n226 = Add(x=w540, y=5) -> (x+y=w555:i32)
                n227 = And(x=w553, y=w551) -> (x .and. y?=w552:bool)
                n228 = Select(t=w555, s=w552, f=w540) -> (s? t:f=w539:i32)
              }
              frame "Lumbares" {
                n229 = Greater Or Equal To 0?(x=w557) -> (x >= 0?=w570:bool)
                n230 = Less Or Equal?(x=w557, y=100) -> (x <= y?=w568:bool)
                n231 = Add(x=w557, y=5) -> (x+y=w572:i32)
                n232 = And(x=w570, y=w568) -> (x .and. y?=w569:bool)
                n233 = Select(t=w572, s=w569, f=w557) -> (s? t:f=w556:i32)
              }
              frame "Dorsales" {
                n234 = Greater Or Equal To 0?(x=w573) -> (x >= 0?=w587:bool)
                n235 = Less Or Equal?(x=w573, y=100) -> (x <= y?=w585:bool)
                n236 = Add(x=w573, y=5) -> (x+y=w589:i32)
                n237 = And(x=w587, y=w585) -> (x .and. y?=w586:bool)
                n238 = Select(t=w589, s=w586, f=w573) -> (s? t:f=w574:i32)
              }
              frame "Trapecio" {
                n239 = Greater Or Equal To 0?(x=w591) -> (x >= 0?=w604:bool)
                n240 = Less Or Equal?(x=w591, y=100) -> (x <= y?=w602:bool)
                n241 = Add(x=w591, y=5) -> (x+y=w606:i32)
                n242 = And(x=w604, y=w602) -> (x .and. y?=w603:bool)
                n243 = Select(t=w606, s=w603, f=w591) -> (s? t:f=w590:i32)
              }
              frame "Pectorales" {
                n244 = Greater Or Equal To 0?(x=w609) -> (x >= 0?=w621:bool)
                n245 = Less Or Equal?(x=w609, y=100) -> (x <= y?=w619:bool)
                n246 = Add(x=w609, y=5) -> (x+y=w623:i32)
                n247 = And(x=w621, y=w619) -> (x .and. y?=w620:bool)
                n248 = Select(t=w623, s=w620, f=w609) -> (s? t:f=w607:i32)
              }
              frame "Biceps" {
                n249 = Greater Or Equal To 0?(x=w624) -> (x >= 0?=w638:bool)
                n250 = Less Or Equal?(x=w624, y=100) -> (x <= y?=w636:bool)
                n251 = Add(x=w624, y=5) -> (x+y=w640:i32)
                n252 = And(x=w638, y=w636) -> (x .and. y?=w637:bool)
                n253 = Select(t=w640, s=w637, f=w624) -> (s? t:f=w625:i32)
              }
              frame "Opcional" {
                n254 = Greater Or Equal To 0?(x=w642) -> (x >= 0?=w655:bool)
                n255 = Less Or Equal?(x=w642, y=100) -> (x <= y?=w653:bool)
                n256 = Add(x=w642, y=5) -> (x+y=w657:i32)
                n257 = And(x=w655, y=w653) -> (x .and. y?=w654:bool)
                n258 = Select(t=w657, s=w654, f=w642) -> (s? t:f=w641:i32)
              }
              frame Default {
              }
            }
          }
          event "Remove Button": Value Change {
            n259 = event-data() -> ()  [unwired: 1 in, 6 out]
            n260 = case shown="\"Isquiotibiales\"" w689 {
              tunnel: w688 -> [w690 w709 w724 w739 w754 w769 w784 w799 w814 w829 w839]
              tunnel: w687 -> [w703 w717 w731 w745 w759 w773 w787 w801 w815 w816 w830]
              tunnel: w686 -> [w702 w716 w730 w744 w758 w772 w786 w800 w802 w821 w831]
              tunnel: w685 -> [w701 w715 w729 w743 w757 w771 w785 w788 w807 w822 w832]
              tunnel: w684 -> [w700 w714 w728 w742 w756 w770 w775 w793 w808 w823 w833]
              tunnel: w683 -> [w699 w713 w727 w741 w755 w760 w779 w794 w809 w824 w834]
              tunnel: w682 -> [w698 w712 w726 w740 w746 w765 w780 w795 w810 w825 w835]
              tunnel: w681 -> [w697 w711 w725 w732 w751 w766 w781 w796 w811 w826 w836]
              tunnel: w680 -> [w696 w710 w718 w737 w752 w767 w782 w797 w812 w827 w837]
              tunnel: w679 -> [w695 w704 w723 w738 w753 w768 w783 w798 w813 w828 w838]
              tunnel: [w703 w717 w731 w745 w759 w773 w787 w801 w815 w817 w830] -> w670
              tunnel: [w702 w716 w730 w744 w758 w772 w786 w800 w803 w821 w831] -> w671
              tunnel: [w701 w715 w729 w743 w757 w771 w785 w789 w807 w822 w832] -> w672
              tunnel: [w700 w714 w728 w742 w756 w770 w774 w793 w808 w823 w833] -> w673
              tunnel: [w699 w713 w727 w741 w755 w761 w779 w794 w809 w824 w834] -> w674
              tunnel: [w698 w712 w726 w740 w747 w765 w780 w795 w810 w825 w835] -> w675
              tunnel: [w697 w711 w725 w733 w751 w766 w781 w796 w811 w826 w836] -> w676
              tunnel: [w696 w710 w719 w737 w752 w767 w782 w797 w812 w827 w837] -> w677
              tunnel: [w695 w705 w723 w738 w753 w768 w783 w798 w813 w828 w838] -> w678
              tunnel: [w691 w709 w724 w739 w754 w769 w784 w799 w814 w829 w839] -> w669
              frame "Cuadriceps" {
                n261 = Greater Than 0?(x=w690) -> (x > 0?=w694:bool)
                n262 = Subtract(x=w690, y=5) -> (x-y=w693:i32)
                n263 = Select(t=w693, s=w694, f=w690) -> (s? t:f=w691:i32)
              }
              frame "Isquiotibiales" {
                n264 = Greater Than 0?(x=w704) -> (x > 0?=w708:bool)
                n265 = Subtract(x=w704, y=5) -> (x-y=w707:i32)
                n266 = Select(t=w707, s=w708, f=w704) -> (s? t:f=w705:i32)
              }
              frame "Gluteos" {
                n267 = Greater Than 0?(x=w718) -> (x > 0?=w722:bool)
                n268 = Subtract(x=w718, y=5) -> (x-y=w721:i32)
                n269 = Select(t=w721, s=w722, f=w718) -> (s? t:f=w719:i32)
              }
              frame "Abdomen" {
                n270 = Greater Than 0?(x=w732) -> (x > 0?=w736:bool)
                n271 = Subtract(x=w732, y=5) -> (x-y=w735:i32)
                n272 = Select(t=w735, s=w736, f=w732) -> (s? t:f=w733:i32)
              }
              frame "Lumbares" {
                n273 = Greater Than 0?(x=w746) -> (x > 0?=w750:bool)
                n274 = Subtract(x=w746, y=5) -> (x-y=w749:i32)
                n275 = Select(t=w749, s=w750, f=w746) -> (s? t:f=w747:i32)
              }
              frame "Dorsales" {
                n276 = Greater Than 0?(x=w760) -> (x > 0?=w764:bool)
                n277 = Subtract(x=w760, y=5) -> (x-y=w763:i32)
                n278 = Select(t=w763, s=w764, f=w760) -> (s? t:f=w761:i32)
              }
              frame "Trapecio" {
                n279 = Greater Than 0?(x=w775) -> (x > 0?=w778:bool)
                n280 = Subtract(x=w775, y=5) -> (x-y=w777:i32)
                n281 = Select(t=w777, s=w778, f=w775) -> (s? t:f=w774:i32)
              }
              frame "Pectorales" {
                n282 = Greater Than 0?(x=w788) -> (x > 0?=w792:bool)
                n283 = Subtract(x=w788, y=5) -> (x-y=w791:i32)
                n284 = Select(t=w791, s=w792, f=w788) -> (s? t:f=w789:i32)
              }
              frame "Biceps" {
                n285 = Greater Than 0?(x=w802) -> (x > 0?=w806:bool)
                n286 = Subtract(x=w802, y=5) -> (x-y=w805:i32)
                n287 = Select(t=w805, s=w806, f=w802) -> (s? t:f=w803:i32)
              }
              frame "Opcional" {
                n288 = Greater Than 0?(x=w816) -> (x > 0?=w820:bool)
                n289 = Subtract(x=w816, y=5) -> (x-y=w819:i32)
                n290 = Select(t=w819, s=w820, f=w816) -> (s? t:f=w817:i32)
              }
              frame Default {
              }
            }
          }
          event "Slider": Value Change {
            n291 = event-data() -> ()  [unwired: 1 in, 6 out]
            n292 = case shown="\"Cuadriceps\"" w842 {
              tunnel: w843 -> [_ w874 w885 w896 w907 w918 w929 w940 w951 w962 w972]
              tunnel: w844 -> [w872 w882 w892 w902 w912 w922 w932 w942 w952 _ w963]
              tunnel: w845 -> [w871 w881 w891 w901 w911 w921 w931 w941 _ w954 w964]
              tunnel: w846 -> [w870 w880 w890 w900 w910 w920 w930 _ w944 w955 w965]
              tunnel: w847 -> [w869 w879 w889 w899 w909 w919 _ w934 w945 w956 w966]
              tunnel: w848 -> [w868 w878 w888 w898 w908 _ w924 w935 w946 w957 w967]
              tunnel: w849 -> [w867 w877 w887 w897 _ w914 w925 w936 w947 w958 w968]
              tunnel: w850 -> [w866 w876 w886 _ w904 w915 w926 w937 w948 w959 w969]
              tunnel: w851 -> [w865 w875 _ w894 w905 w916 w927 w938 w949 w960 w970]
              tunnel: w852 -> [w864 _ w884 w895 w906 w917 w928 w939 w950 w961 w971]
              tunnel: [w872 w882 w892 w902 w912 w922 w932 w942 w952 w953 w963] -> w853
              tunnel: [w871 w881 w891 w901 w911 w921 w931 w941 w943 w954 w964] -> w854
              tunnel: [w870 w880 w890 w900 w910 w920 w930 w933 w944 w955 w965] -> w855
              tunnel: [w869 w879 w889 w899 w909 w919 w923 w934 w945 w956 w966] -> w856
              tunnel: [w868 w878 w888 w898 w908 w913 w924 w935 w946 w957 w967] -> w857
              tunnel: [w867 w877 w887 w897 w903 w914 w925 w936 w947 w958 w968] -> w858
              tunnel: [w866 w876 w886 w893 w904 w915 w926 w937 w948 w959 w969] -> w859
              tunnel: [w865 w875 w883 w894 w905 w916 w927 w938 w949 w960 w970] -> w860
              tunnel: [w864 w873 w884 w895 w906 w917 w928 w939 w950 w961 w971] -> w861
              tunnel: [w863 w874 w885 w896 w907 w918 w929 w940 w951 w962 w972] -> w862
              tunnel: "Slider" -> [w863 w873 w883 w893 w903 w913 w923 w933 w943 w953 _]
              frame "Cuadriceps" {
              }
              frame "Isquiotibiales" {
              }
              frame "Gluteos" {
              }
              frame "Abdomen" {
              }
              frame "Lumbares" {
              }
              frame "Dorsales" {
              }
              frame "Trapecio" {
              }
              frame "Pectorales" {
              }
              frame "Biceps" {
              }
              frame "Opcional" {
              }
              frame Default {
              }
            }
          }
          event "Stop": Value Change {
            n293 = event-data() -> ()  [unwired: 1 in, 6 out]
          }
          event "Back": Value Change {
            n294 = event-data() -> ()  [unwired: 1 in, 6 out]
          }
          event "Reset": Value Change {
            w1000 = 0 ("Slider")
            n295 = event-data() -> ()  [unwired: 1 in, 6 out]
          }
          event "Help": Value Change {
            n296 = event-data() -> ()  [unwired: 1 in, 6 out]
          }
          event "Impulso": Value Change {
            n297 = event-data() -> ()  [unwired: 1 in, 6 out]
            n298 = call "Impulso.vi"() -> ("Parametros"=w1016:cluster{i32, i32, i32, i32, i32, dbl})  [unwired: 2 in]
          }
          event "Start": Value Change {
            n299 = event-data() -> ()  [unwired: 1 in, 6 out]
            "Boolean" <- "Start"
          }
        }
      }
    }
    frame Error {
    }
  }
  "error out" <- w8
  "Message" <- w7
